vi "Apply Signal Names.vi"(8 "error in":errorcluster, 11 "DIG_IO in":refnum<class "DIG_IO.lvclass">) -> (0 "error out":errorcluster, 3 "DIG_IO out":refnum<class "DIG_IO.lvclass">)   [LabVIEW 2019, in "DIG_IO.lvlib" / "DIG_IO.lvclass"]
uses:
  Library/DIG_IO.lvclass
  C:/Users/Public/Documents/Development/builds/Tools/Config.lvlibp/Config.lvclass
  Library/DIG_IO.lvclass/DIG_IO.ctl
  builds/Tools/Config.lvlibp/Accessors/Read Device Signals.vi
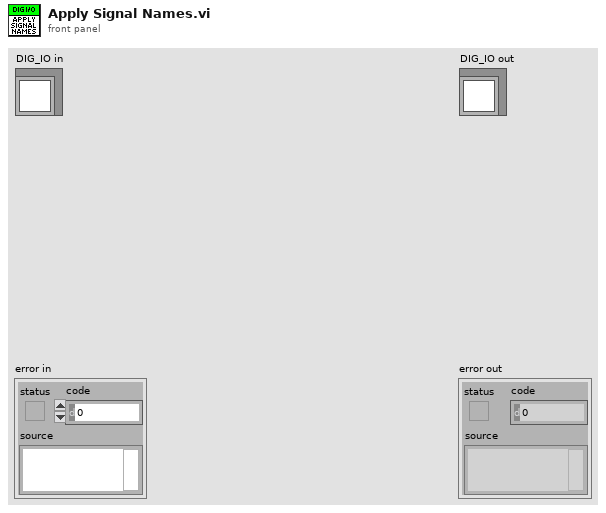
[diagram p1: front panel]
types:
  T1 = enum8{"Enabled", "Disabled", "Disabled and Grayed Out"}
  T2 = enum8{"Enabled", "Disabled", "Disabled and Grayed Out"}[]
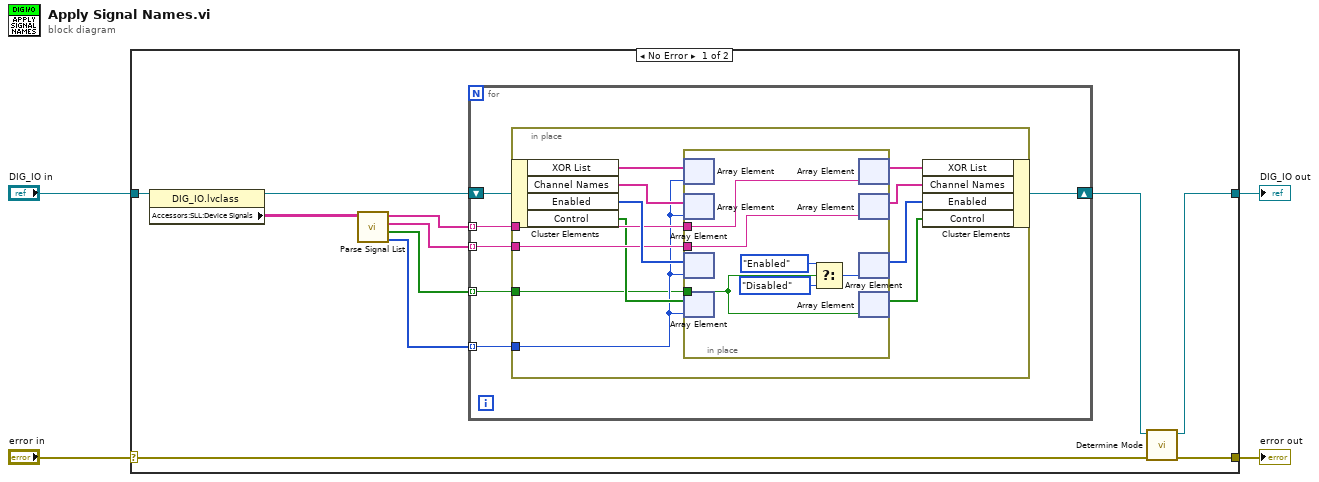
[diagram p0: block diagram]
diagram:
  n1 = case shown="No Error" "error in" {
    selector: "error in" -> [w7 w41]
    tunnel: [w5 w41] -> w3
    tunnel: [w6 w40] -> w1
    tunnel: "DIG_IO in" -> [w15 w40]
    frame No Error {
      n2 = property class="DIG_IO.lvclass"(reference=w15) -> (reference out=w13:refnum<class "DIG_IO.lvclass">, "Accessors:SLL:Device Signals"=w10:string[][])  [unwired: 1 in, 1 out]
      n3 = call "Parse Signal List.vi"("Signal List"=w10) -> ("Pins"=w11:i32[], "Control?"=w12:bool[], "Names"=w14:string[], "XOR List"=w9:string[])  [unwired: 7 in]
      n4 = for {
        shift-right: [w19] -> w8
        shift-left: w13 -> [w20]
        tunnel: w14 -> [w21] mode=indexing
        tunnel: w12 -> [w18] mode=indexing
        tunnel: w11 -> [w17] mode=indexing
        tunnel: w9 -> [w16] mode=indexing
        n5 = in-place {
          in-place-border: w21 -> [w27]
          in-place-border: w18 -> [w23]
          in-place-border: w17 -> [w24]
          in-place-border: w16 -> [w26]
          n6 = in-place-cluster #1(w20) -> ("XOR List"=w32:string[], "Channel Names"=w31:string[], "Enabled"=w30:T2, "Control"=w25:bool[])
          n7 = in-place {
            in-place-border: w27 -> [w38]
            in-place-border: w26 -> [w39]
            in-place-border: w23 -> [w34]
            n8 = in-place-array #2(w32, w24) -> ()  [unwired: 1 out]
            n9 = in-place-array #3(w31, w24) -> ()  [unwired: 1 out]
            n10 = in-place-array #4(w30, w24) -> ()  [unwired: 1 out]
            n11 = in-place-array #5(w25, w24) -> ()  [unwired: 1 out]
            n12 = Select(t=T1."Enabled" ("element"), s=w34, f=T1."Disabled" ("element")) -> (s? t:f=w35:T1)
            n13 = in-place-array #2(w39) -> (w33:string[])  [unwired: 1 out]
            n14 = in-place-array #3(w38) -> (w28:string[])  [unwired: 1 out]
            n15 = in-place-array #4(w35) -> (w29:T2)  [unwired: 1 out]
            n16 = in-place-array #5(w34) -> (w22:bool[])  [unwired: 1 out]
          }
          n17 = in-place-cluster #1("XOR List"=w33, "Channel Names"=w28, "Enabled"=w29, "Control"=w22) -> (w19:refnum<class "DIG_IO.lvclass">)
        }
      }
      n18 = call "Determine Mode.vi"("error in (no error)"=w7, "DIG_IO in"=w8) -> ("error out"=w5:errorcluster, "DIG_IO out"=w6:refnum<class "DIG_IO.lvclass">)  [unwired: 8 in]
    }
    frame Error {
    }
  }
  "error out" <- w3
  "DIG_IO out" <- w1
